vi "FontDialog.vi"(8 "错误输入（无错误）":errorcluster, 10 "ShowEffects":bool, 11 "ShowColor":bool) -> (0 "错误输出":errorcluster, 3 "ShowDialog":i32(ring) items=["None", "OK", "Cancel", "Abort", "Retry", "Ignore", "Yes", "No"])   [LabVIEW 2012]
uses:
  Font.ctl
  System.Windows.Forms
  System.Drawing
panel:
  out "Font":T1 {"Unit" items=["World", "Display", "Pixel", "Point", "Inch", "Document", "Millimeter"]; "Style" items=["Regular"=0, "Bold"=1, "Italic"=2, "Underline"=4, "Strikeout"=8]}
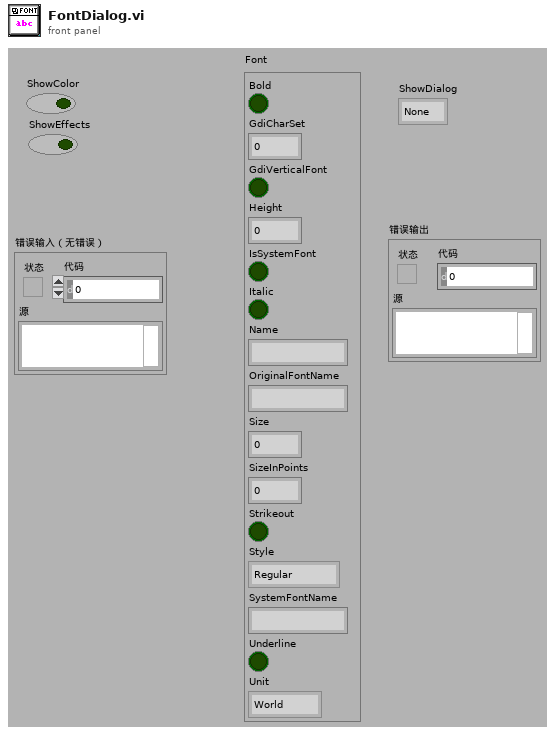
[diagram p1: front panel]
types:
  T1 = typedef "Font.ctl" = cluster{"Bold":bool, "GdiCharSet":u8, "GdiVerticalFont":bool, "Height":i32, "IsSystemFont":bool, "Italic":bool, "Name":string, "OriginalFontName":string, "Size":sgl, "SizeInPoints":sgl, "Strikeout":bool, "Style":i32, "SystemFontName":string, "Underline":bool, "Unit":i32}
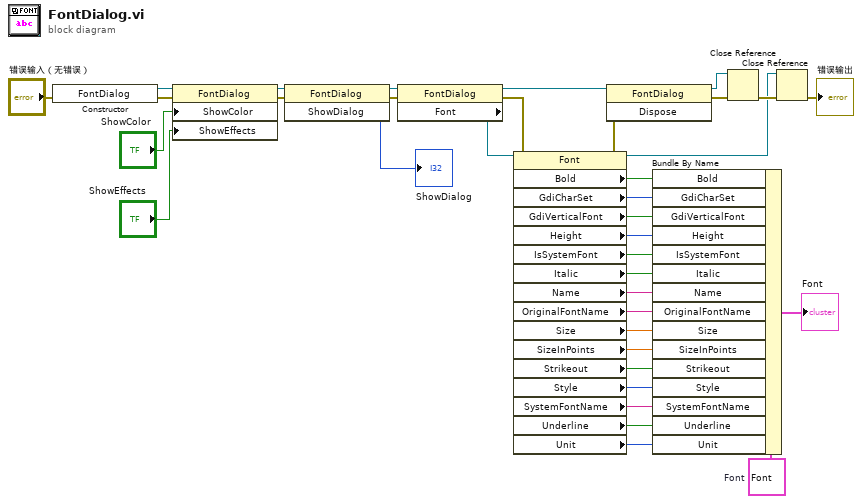
[diagram p0: block diagram]
diagram:
  w26 = T1 {"Bold"=FALSE, "GdiCharSet"=0, "GdiVerticalFont"=FALSE, "Height"=0, "IsSystemFont"=FALSE, "Italic"=FALSE, "Name"="", "OriginalFontName"="", "Size"=0.0, "SizeInPoints"=0.0, "Strikeout"=FALSE, "Style"=0, "SystemFontName"="", "Underline"=FALSE, "Unit"=0}  # Font
  n1 = constructor class="FontDialog"(error in="错误输入（无错误）") -> (reference out=w35:refnum<k24>, error out=w36:errorcluster)  [unwired: 2 in, 1 out]
  n2 = property class="FontDialog"(reference=w35, error in=w36, "ShowColor"="ShowColor", "ShowEffects"="ShowEffects") -> (reference out=w32:refnum<k24>, error out=w31:errorcluster)
  n3 = invoke class="FontDialog" method="ShowDialog"(reference=w32, error in=w31) -> (reference out=w29:refnum<k24>, error out=w28:errorcluster, "ShowDialog"=→"ShowDialog":i32)  [unwired: 1 in]
  n4 = property class="FontDialog"(reference=w29, error in=w28) -> (reference out=w9:refnum<k24>, error out=w7:errorcluster, "Font"=w27:refnum<k24>)
  n5 = property class="Font"(reference=w27, error in=w7) -> (reference out=w3:refnum<k24>, error out=w6:errorcluster, "Bold"=w24:bool, "GdiCharSet"=w23:u8, "GdiVerticalFont"=w22:bool, "Height"=w21:i32, "IsSystemFont"=w20:bool, "Italic"=w19:bool, "Name"=w18:string, "OriginalFontName"=w17:string, "Size"=w16:sgl, "SizeInPoints"=w15:sgl, "Strikeout"=w14:bool, "Style"=w13:i32, "SystemFontName"=w12:string, "Underline"=w11:bool, "Unit"=w10:i32)
  n6 = invoke class="FontDialog" method="Dispose"(reference=w9, error in=w6) -> (reference out=w4:refnum<k24>, error out=w5:errorcluster)  [unwired: 1 in, 1 out]
  n7 = Bundle By Name(cluster=w26, "Bold"=w24, "GdiCharSet"=w23, "GdiVerticalFont"=w22, "Height"=w21, "IsSystemFont"=w20, "Italic"=w19, "Name"=w18, "OriginalFontName"=w17, "Size"=w16, "SizeInPoints"=w15, "Strikeout"=w14, "Style"=w13, "SystemFontName"=w12, "Underline"=w11, "Unit"=w10) -> (→"Font":T1)
  n8 = Close Reference(reference=w4, error in (no error)=w5) -> (error out=w8:errorcluster)
  n9 = Close Reference(reference=w3, error in (no error)=w8) -> (error out=→"错误输出":errorcluster)
